vi "String to different type.vi"(11 "Value":string) -> (3 "Value":T1)   [LabVIEW 2015, in "SQLite.lvclass"]
uses:
  SQLite.lvclass
  Control/value Type.ctl
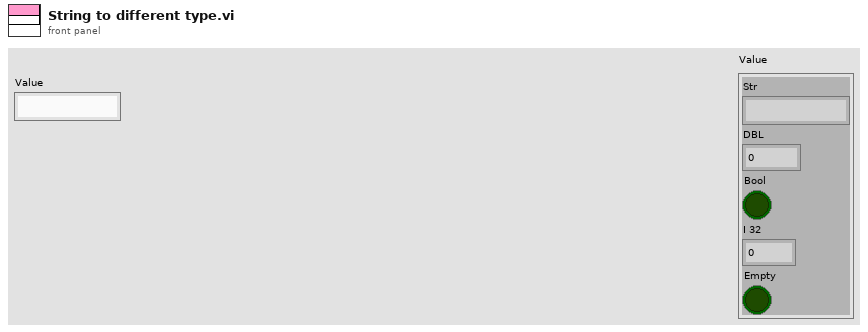
[diagram p1: front panel]
types:
  T1 = typedef "SQLite.lvclass/value Type.ctl" = cluster{"Str":string, "DBL":dbl, "Bool":bool, "I 32":i32, "Empty":bool}
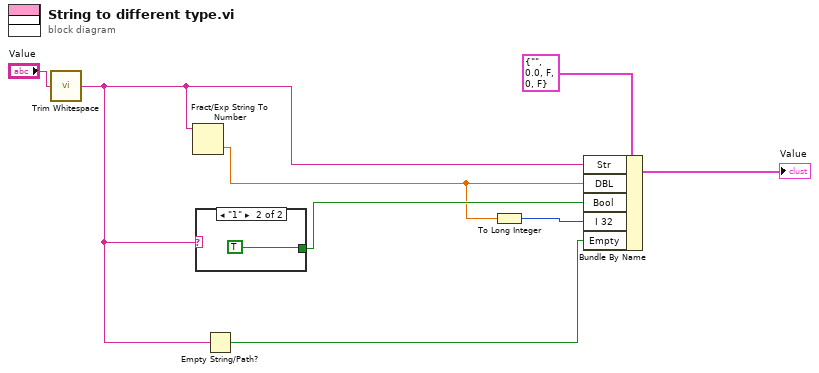
[diagram p0: block diagram]
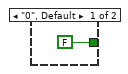
[diagram p2: hidden frame]
diagram:
  n1 = call <vilib>:"Trim Whitespace.vi"("string"="Value") -> ("trimmed string"=w2:string)  [unwired: 1 in]
  n2 = Fract/Exp String To Number(string=w2) -> (number=w4:dbl)  [unwired: 3 in, 1 out]
  n3 = case shown="\"1\"" w2 {
    tunnel: [FALSE ("Boolean") TRUE ("Boolean")] -> w5
    frame "0", Default {
    }
    frame "1" {
    }
  }
  n4 = Empty String/Path?(string/path=w2) -> (empty?=w1:bool)
  n5 = To Long Integer(number=w4) -> (32bit integer=w3:i32)
  n6 = Bundle By Name(cluster=T1 {"Str"="", "DBL"=0.0, "Bool"=FALSE, "I 32"=0, "Empty"=FALSE} ("Value"), "Str"=w2, "DBL"=w4, "Bool"=w5, "I 32"=w3, "Empty"=w1) -> (→"Value":T1)
